vi "Get Panel Hwnd.vi"(8 "error in (no error)":errorcluster, 11 "Panel":refnum<k24>(container)) -> (0 "error out":errorcluster, 2 "HWND":u64, 3 "Container reference out":refnum<k24>)   [LabVIEW 2016, in "LV MDI.lvclass"]
uses:
  LV MDI.lvclass
  System.Windows.Forms
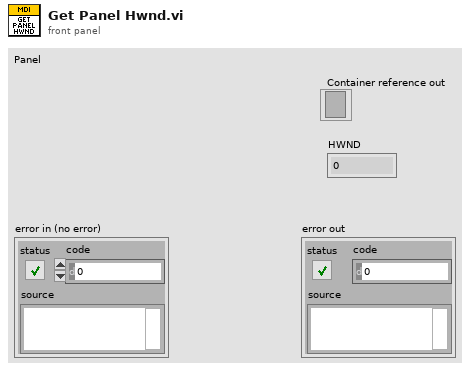
[diagram p1: front panel]
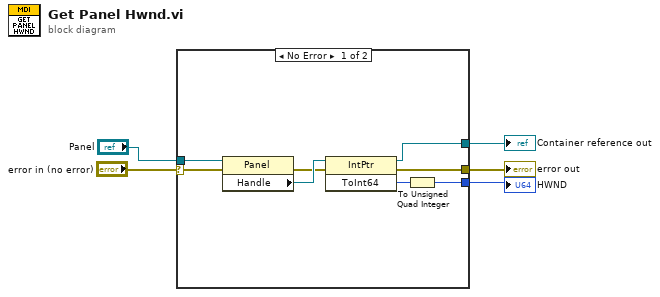
[diagram p0: block diagram]
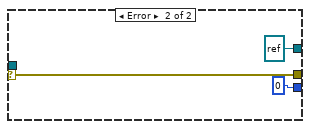
[diagram p2: hidden frame]
diagram:
  n1 = case shown="No Error" "error in (no error)" {
    selector: "error in (no error)" -> [w8 w15]
    tunnel: [w11 refnum<k24> refnum ("Handle")] -> w5
    tunnel: [w10 w15] -> w4
    tunnel: [w6 i64 0 ("ToInt64")] -> w3
    tunnel: "Panel" -> [w7 _]
    frame No Error {
      n2 = property class="Panel"(reference=w7, error in=w8) -> (error out=w12:errorcluster, "Handle"=w13:refnum<k24>)  [unwired: 1 out]
      n3 = invoke class="IntPtr" method="ToInt64"(reference=w13, error in=w12) -> (reference out=w11:refnum<k24>, error out=w10:errorcluster, "ToInt64"=w9:i64)  [unwired: 1 in]
      n4 = To Unsigned Quad Integer(1:w9) -> (0:w6:u64)
    }
    frame Error {
    }
  }
  "Container reference out" <- w5
  "error out" <- w4
  "HWND" <- w3
